vi "Waveform - Get Subset.vi"() -> ()   [LabVIEW 2023]
doc: "Shows how to get a subset of a waveform."
uses:
  <vilib>/Waveform/WDTOps.llb/WDT Get Waveform Subset DBL.vi
panel:
  in  "Duration":dbl=30.0
  in  "Start Index":dbl=35.0
  out "Waveforms":waveform(dbl)[](graph)
  # "Overview: Demonstrates how to retrieve a subset of a waveform with the Get Waveform Subset VI.\nInstructions:\n1. Select a Start Index value and a Duration.\n2. Run the VI. The specified subset of the waveform will be displayed as the Subset Waveform plot over the original waveform."
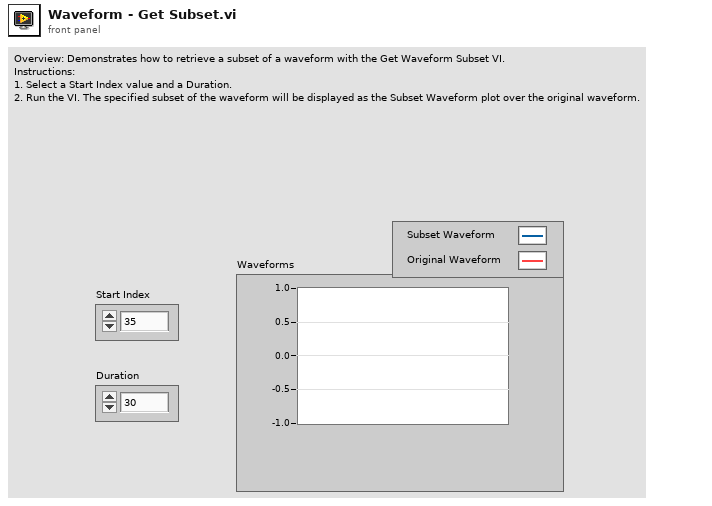
[diagram p1: front panel]
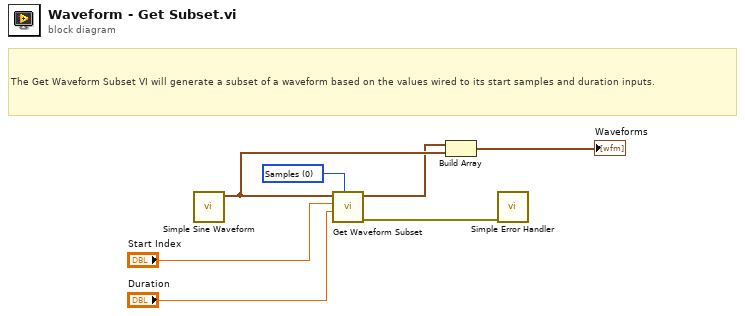
[diagram p0: block diagram]
diagram:
  w3 = u16 0 items=["Samples", "Relative Time"] ("start/duration format")
  # "The Get Waveform Subset VI will generate a subset of a waveform based on the values wired to its start samples and duration inputs."
  n1 = call "Simple Sine Waveform.vi"() -> ("sine waveform"=w7:waveform(dbl))  [unwired: 11 in]
  n2 = call-poly <vilib>:"Get Waveform Subset.vi"("start/duration format"=w3, "duration"="Duration", "start samples/time"="Start Index", "waveform in"=w7) -> ("error out"=w2:errorcluster, "waveform out"=w4:waveform(dbl))  [unwired: 2 in, 2 out]
  n3 = Build Array(w4, w7) -> (→"Waveforms":waveform(dbl)[])
  n4 = call <vilib>:"Simple Error Handler.vi"("error in (no error)"=w2) -> ()  [unwired: 4 in, 5 out]
